vi "GetRotatedPosition.vi"(8 "theta":dbl, 10 "Y":dbl, 11 "X":dbl) -> (2 "Y'":dbl, 3 "X'":dbl)   [LabVIEW 2018]
uses:
  <vilib>/Analysis/coordinate.llb/2D Cartesian Coordinate Rotation (Scalar).vi
  <vilib>/Analysis/NI_AALPro.lvlib
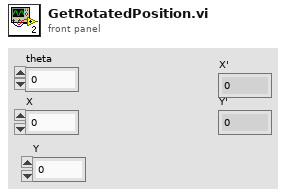
[diagram p1: front panel]
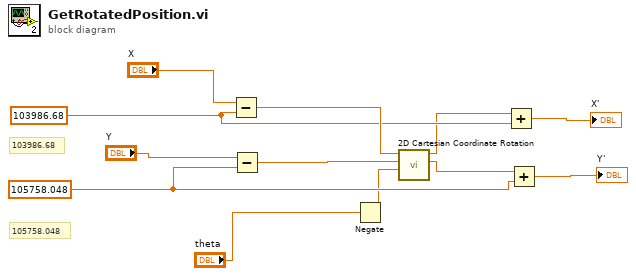
[diagram p0: block diagram]
diagram:
  w7 = 105758.048 ("y")
  w8 = 103986.68 ("y")
  # "103986.68"
  # "105758.048"
  n1 = Subtract(x="X", y=w8) -> (x-y=w10:dbl)
  n2 = Subtract(x="Y", y=w7) -> (x-y=w9:dbl)
  n3 = Negate(x="theta") -> (-x=w2:dbl)
  n4 = call-poly <vilib>:"2D Cartesian Coordinate Rotation.vi"("theta"=w2, "y"=w9, "x"=w10) -> ("y out"=w6:dbl, "x out"=w5:dbl)  [unwired: 6 in, 1 out]
  n5 = Add(x=w5, y=w8) -> (x+y=→"X'":dbl)
  n6 = Add(x=w6, y=w7) -> (x+y=→"Y'":dbl)
